vi "ToggleAxis.vi"(11 "FPGA VI Reference Out":refnum<k20>) -> ()   [LabVIEW 2009]
uses:
  <vilib>/rvi/interface/nirviReadWriteControl/nirviReadWriteControl.xnode
  FPGA_Control/AOD Control (FPGA).vi
  FPGA_Control/FPGA Bitfiles/AOD Control.lvproj_PXI-7954R_AOD Control (FPGA)~D2.lvbitx
panel:
  out "Phase":bool
  in  "Pause (ms)":dbl=1000.0
  in  "Toggle":bool
  in  "stop":bool
  in  "Center Frequencies":T1={"XHP"=805306367, "XLP"=805306367, "YHP"=858993459, "YLP"=858993459} {"XHP" format="%x"; "XLP" format="%x"; "YHP" format="%x"; "YLP" format="%x"}
  in  "Delta":T1 {"XHP" format="%x"; "XLP" format="%x"; "YHP" format="%x"; "YLP" format="%x"}
  out "Setting":T1
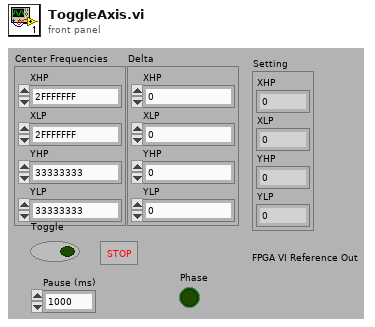
[diagram p1: front panel]
types:
  T1 = cluster{"XHP":i32, "XLP":i32, "YHP":i32, "YLP":i32}
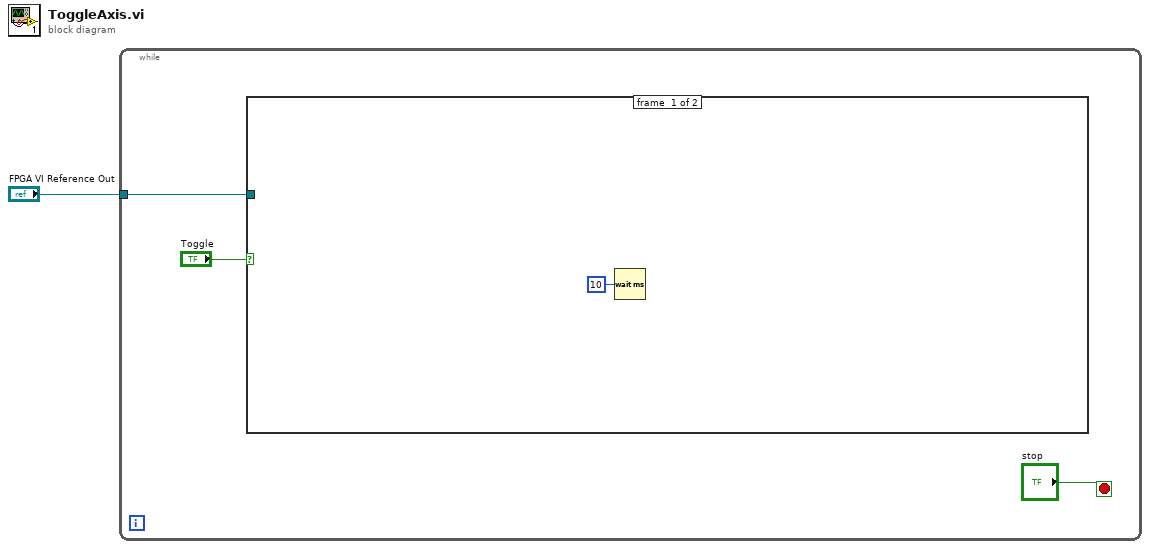
[diagram p0: block diagram]
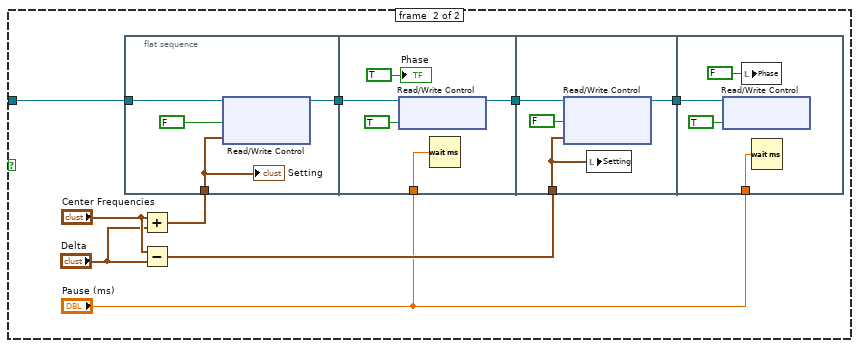
[diagram p2: hidden frame]
diagram:
  n1 = while {
    tunnel: "FPGA VI Reference Out" -> [w3]
    stop <- "stop" stop-if-true
    n2 = case shown="True" "Toggle" {
      tunnel: w3 -> [_ w11]
      frame #0 {
        n3 = Wait (ms)(milliseconds to wait=u32 10) -> ()  [unwired: 1 out]
      }
      frame #1 {
        n4 = flat-sequence {
          tunnel: w11 -> [w17]
          tunnel: w12 -> [w15]
          tunnel: [w16] -> w14
          tunnel: w14 -> [w28]
          tunnel: [w27] -> w13
          tunnel: "Pause (ms)" -> [w26]
          tunnel: w13 -> [w38]
          tunnel: w8 -> [w37]
          tunnel: [w36] -> w7
          tunnel: w7 -> [w48]
          tunnel: "Pause (ms)" -> [w47]
          frame #0 {
            n5 = xnode "Read/Write Control"("FPGA VI Reference In"=w17, "SetCoordinate"=FALSE, "Coordinate"=w15) -> ("FPGA VI Reference Out"=w16:refnum<k20>)  [unwired: 1 in, 1 out]
            "Setting" <- w15
          }
          frame #1 {
            n6 = xnode "Read/Write Control"("FPGA VI Reference In"=w28, "SetCoordinate"=TRUE) -> ("FPGA VI Reference Out"=w27:refnum<k20>)  [unwired: 1 in, 1 out]
            n7 = Wait (ms)(milliseconds to wait=w26) -> ()  [unwired: 1 out]
            "Phase" <- TRUE ("Phase")
          }
          frame #2 {
            n8 = xnode "Read/Write Control"("FPGA VI Reference In"=w38, "SetCoordinate"=FALSE, "Coordinate"=w37) -> ("FPGA VI Reference Out"=w36:refnum<k20>)  [unwired: 1 in, 1 out]
            n9 = local write "Setting"(w37) -> ()
          }
          frame #3 {
            n10 = xnode "Read/Write Control"("FPGA VI Reference In"=w48, "SetCoordinate"=TRUE) -> ()  [unwired: 1 in, 2 out]
            n11 = local write "Phase"(FALSE ("Phase")) -> ()
            n12 = Wait (ms)(milliseconds to wait=w47) -> ()  [unwired: 1 out]
          }
        }
        n13 = Add(x="Center Frequencies", y="Delta") -> (x+y=w12:T1)
        n14 = Subtract(x="Center Frequencies", y="Delta") -> (x-y=w8:T1)
      }
    }
  }
